vi "LVFunction_Imop_GetHardwareConfig.vi"(0 "WFS_setupfile_IN":path, 11 "error in":errorcluster) -> (4 "WFS_setupfile_OUT":path, 6 "HardwareOptions":T1, 15 "error out":errorcluster)   [LabVIEW 2018]
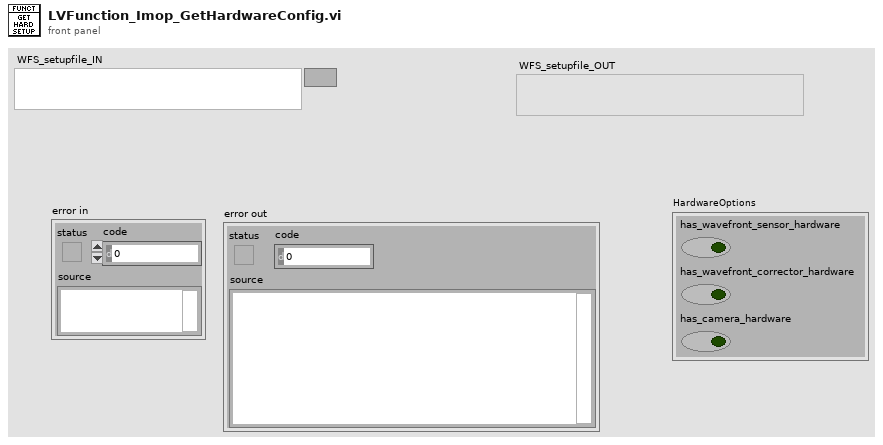
[diagram p1: front panel]
types:
  T1 = cluster{"has_wavefront_sensor_hardware":bool, "has_wavefront_corrector_hardware":bool, "has_camera_hardware":bool}
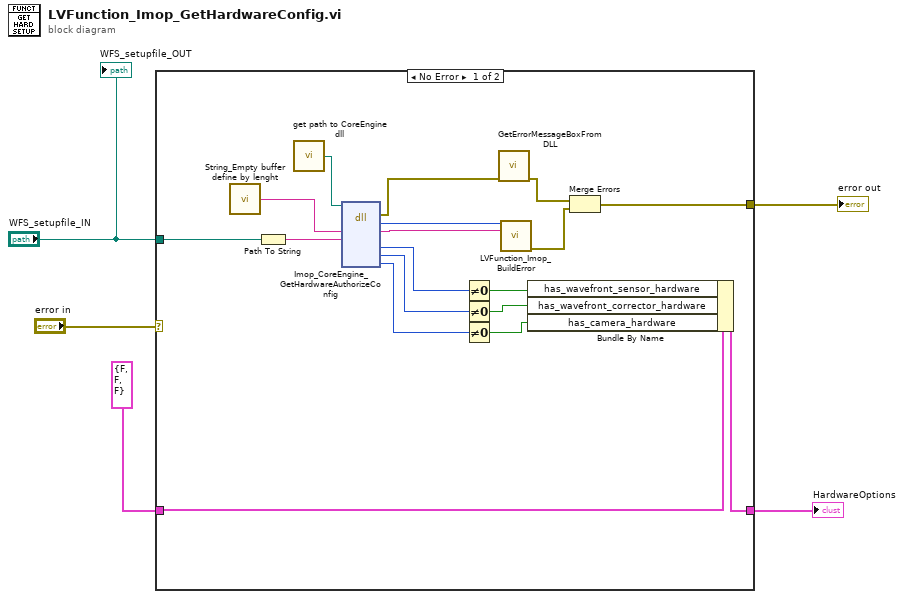
[diagram p0: block diagram]
diagram:
  n1 = case shown="No Error" "error in" {
    selector: "error in" -> [_ w25]
    tunnel: [w16 w25] -> w4
    tunnel: "WFS_setupfile_IN" -> [w15 _]
    tunnel: T1 {"has_wavefront_sensor_hardware"=FALSE, "has_wavefront_corrector_hardware"=FALSE, "has_camera_hardware"=FALSE} ("Cluster") -> [w10 w24]
    tunnel: [w6 w24] -> w2
    frame No Error {
      n2 = call "String_Empty buffer define by lenght.vi"() -> ("Empty buffer"=w17:string)  [unwired: 1 in]
      n3 = Path To String(path=w15) -> (string=w14:string)
      n4 = call "get path to CoreEngine dll.vi"() -> ("path to wavekit library"=w20:path)  [unwired: 14 in, 1 out]
      n5 = dll-call lib="D:/soft/HASO_v3/SVN_trunk/ImOpCoreEngine4_LV2011/DLLs/c_interface_vc100.dll" fn="Imop_CoreEngine_GetHardwareAuthorizeConfig"(path in=w20, "message"=w17, "config_file_path"=w14) -> (error out=w21:errorcluster, "return type"=w19:i32, "message"=w18:string, "has_wavefront_sensor_hardware"=w13:u8, "has_wavefront_corrector_hardware"=w11:u8, "has_camera_hardware"=w12:u8)  [unwired: 6 in, 1 out]
      n6 = Not Equal To 0?(x=w13) -> (x != 0?=w9:bool)
      n7 = Not Equal To 0?(x=w11) -> (x != 0?=w8:bool)
      n8 = Not Equal To 0?(x=w12) -> (x != 0?=w7:bool)
      n9 = call "GetErrorMessageBoxFromDLL.vi"("error IN"=w21) -> ("error OUT"=w22:errorcluster)  [unwired: 10 in]
      n10 = call "LVFunction_Imop_BuildError.vi"("code"=w19, "String to Prepend to source (\"\")"=w18) -> ("error out"=w23:errorcluster)  [unwired: 13 in]
      n11 = Bundle By Name(cluster=w10, "has_wavefront_sensor_hardware"=w9, "has_wavefront_corrector_hardware"=w8, "has_camera_hardware"=w7) -> (w6:T1)
      n12 = Merge Errors(w22, w23) -> (w16:errorcluster)
    }
    frame Error {
    }
  }
  "error out" <- w4
  "HardwareOptions" <- w2
  "WFS_setupfile_OUT" <- "WFS_setupfile_IN"
